vi "Get Resource Type.vi"(11 "I2C in":refnum<class "I2C.lvclass">) -> (2 "Resource Type":string)   [LabVIEW 2020, in "CTI.lvlib" / "I2C.lvclass"]
uses:
  I2C.lvclass
  I2C.lvclass/I2C.ctl
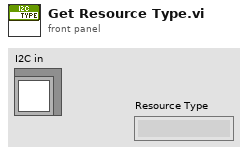
[diagram p1: front panel]
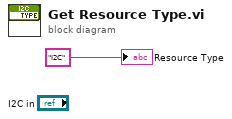
[diagram p0: block diagram]
diagram:
  "Resource Type" <- "I2C" ("Resource Type")
